vi "TCP SEND SWITCH.vi"   [LabVIEW 2014]
uses:
  <vilib>/Platform/TimedLoop/XDataNode/wakeup.ctl
  <vilib>/Platform/TimedLoop/XDataNode/XDNodeRunTimeDep.lvlib
  <vilib>/Platform/TimedLoop/XDataNode/nitl_modes.ctl
  <vilib>/Platform/TimedLoop/XDataNode/timing_clust.ctl
  <vilib>/Platform/TimedLoop/XDataNode/XDataNode.xnode
types:
  T1 = typedef "XDNodeRunTimeDep.lvlib/timing_clust.ctl" = cluster{"Expected End [f-1]":u64, "Actual End [f-1]":u64, "Finished Late? [f-1]":bool, "Expected End [i-1]":u64, "Actual End [i-1]":u64, "Finished Late? [i-1]":bool, "Expected Start [i]":u64, "Actual Start [i]":u64, "Expected Start [f]":u64, "Actual Start [f]":u64, "Source Name":string, "Structure Name":string, "Period":i64, "Deadline":i64, "Offset":i64, "Start":i64, "Priority":i32, "Timeout":i32, "Mode":T2, "Wakeup Reason":T3, "Error":errorcluster, "Source Type":string, "Secondary Source Type":string, "Global End Time":u64, "Global Start Time":u64, "Frame Duration":u64, "Iteration Duration":u64, "Assigned CPU":i32, "I/O Scan Engine Mode":u32}
  T2 = typedef "XDNodeRunTimeDep.lvlib/nitl_modes.ctl" = enum32{"No Change", "Process missed periods, maintain original phase", "Discard missed periods, maintain original phase", "Process missed periods, ignore original phase", "Discard missed periods, ignore original phase"}
  T3 = typedef "XDNodeRunTimeDep.lvlib/wakeup.ctl" = enum32{"Normal", "Aborted", "Asynchronous wakeup", "Timing source error", "Timed loop error", "Timeout"}
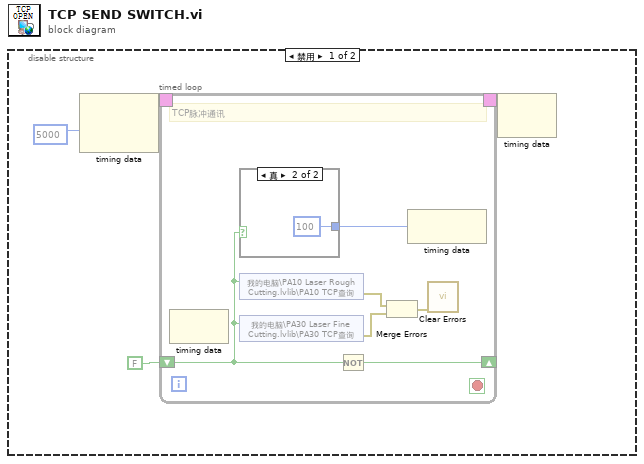
[diagram p0: block diagram]
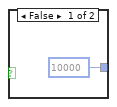
[diagram p2: hidden frame]
diagram:
  n1 = disable-structure shown="禁用" {
    frame Disabled {
      n2 = node-c288(i64 5000 ("周期")) -> (w4:T1)  [unwired: 1 in]
      n3 = timed-loop {
        timing: w4 -> [_]
        timing-out: [_] -> w3
        shift-right: [w10] -> _
        shift-left: FALSE -> [w9]
        stop <- _ stop-if-true
        # "TCP脉冲通讯"
        n4 = node-c288() -> ()  [unwired: 1 in, 1 out]
        n5 = case shown="真" w9 {
          tunnel: [i64 10000 ("期限") i64 100 ("期限")] -> w8
          frame False {
          }
          frame True {
          }
        }
        n6 = shared-variable "我的电脑\\PA10 Laser Rough Cutting.lvlib\\PA10 TCP查询"(w9) -> (error out=w7:errorcluster)  [unwired: 1 in]
        n7 = shared-variable "我的电脑\\PA30 Laser Fine Cutting.lvlib\\PA30 TCP查询"(w9) -> (error out=w6:errorcluster)  [unwired: 1 in]
        n8 = Not(x=w9) -> (.not. x?=w10:bool)
        n9 = Merge Errors(w7, w6) -> (w5:errorcluster)
        n10 = node-c288(w8) -> ()  [unwired: 1 out]
        n11 = call <vilib>:"Clear Errors.vi"("error in (no error)"=w5) -> ()  [unwired: 5 in, 2 out]
      }
      n12 = node-c288(w3) -> ()  [unwired: 1 out]
    }
    frame Enabled {
    }
  }
